vi "Mask and Limit Testing of XY Graph.vi"() -> ()   [LabVIEW 2023]
doc: "This example demonstrates how to create mask for XY graph. The VI checks if the input signal points are in or out of boundary. If any input signal points go beyond boundary, they will be marked in red. You can modify the boundary points that define a polygon and reset them."
uses:
  <vilib>/Analysis/NI_AALBase.lvlib
panel:
  out "XY Graph":cluster{"X":dbl[], "Y":dbl[]}[](graph)
  in  "Boundary":cluster{"X":dbl[], "Y":dbl[]}={"X"=[-0.6, 0.2, 1.0, 0.6, 0.0, -1.0], "Y"=[-1.0, -0.4, -0.6, 1.0, 0.4, 0.8]}
  in  "Reset Boundary":bool
  in  "stop":bool
  # "Overview: Demonstrates how to create a mask for an XY Graph. \nRequirements: LabVIEW Full Development System\nInstructions: \n1. Run the VI.\n2. Insert, delete or modify the boundary points. Click Reset Boundary to reset them.\n3. Click Stop to stop the VI."
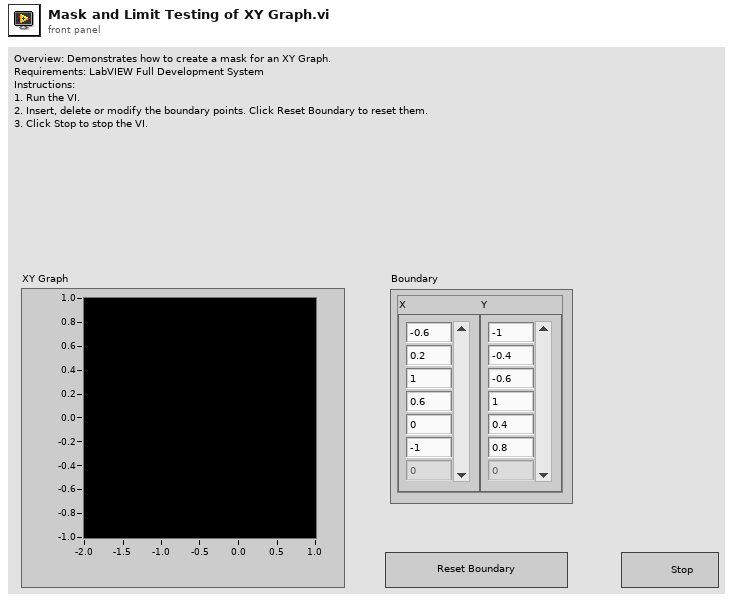
[diagram p1: front panel]
types:
  T1 = cluster{"Sinusoidal Pattern":dbl[], "Sinusoidal Pattern":dbl[]}
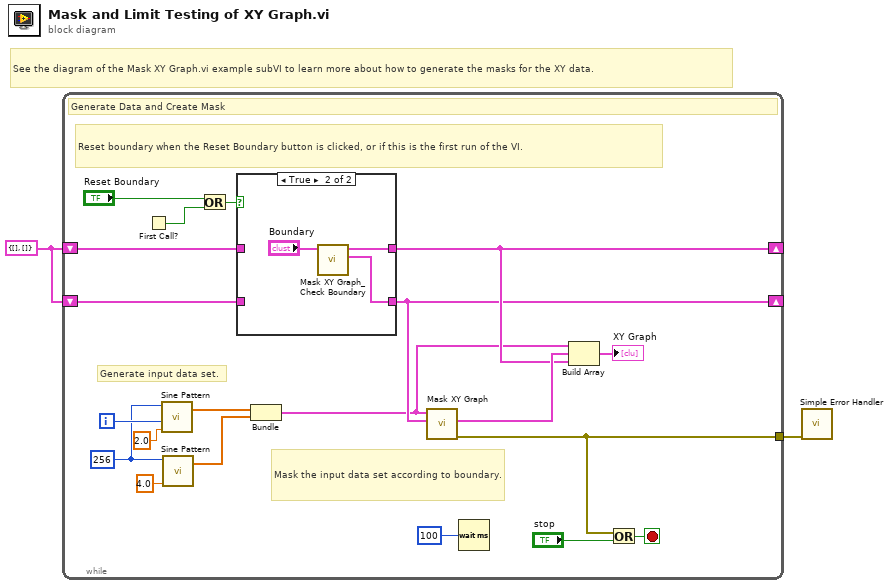
[diagram p0: block diagram]
diagram:
  w1 = cluster{"X":dbl[], "Y":dbl[]} {"X"=[], "Y"=[]} ("Closed Boundary")
  # "See the diagram of the Mask XY Graph.vi example subVI to learn more about how to generate the masks for the XY data."
  n1 = while {
    shift-right: [w17] -> _
    shift-left: w1 -> [w20]
    shift-right: [w16] -> _
    shift-left: w1 -> [w15]
    tunnel: [w5] -> w2
    i -> [w12]
    stop <- w6 stop-if-true
    w9 = 256 ("samples")
    # "Reset boundary when the Reset Boundary button is clicked, or if this is the first run of the VI."
    # "Mask the input data set according to boundary."
    # "Generate input data set."
    # "Generate Data and Create Mask"
    n2 = First Call?() -> (First Call?: T/F=w3:bool)
    n3 = call <vilib>:"Sine Pattern.vi"("cycles"=2.0, "phase(degrees)"=w12, "samples"=w9) -> ("Sinusoidal Pattern"=w11:dbl[])  [unwired: 1 in, 1 out]
    n4 = call <vilib>:"Sine Pattern.vi"("cycles"=4.0, "samples"=w9) -> ("Sinusoidal Pattern"=w10:dbl[])  [unwired: 2 in, 1 out]
    n5 = Or(x="Reset Boundary", y=w3) -> (x .or. y?=w4:bool)
    n6 = case shown="True" w4 {
      tunnel: w20 -> [w24 _]
      tunnel: [w23 w25] -> w16
      tunnel: [w24 w26] -> w17
      tunnel: w15 -> [w23 _]
      frame False {
      }
      frame True {
        n7 = call "Mask XY Graph_Check Boundary.vi"("Boundary"="Boundary") -> ("Open Boundary"=w25:cluster{"X":dbl[], "Y":dbl[]}, "Closed Boundary"=w26:cluster{"X":dbl[], "Y":dbl[]})  [unwired: 9 in]
      }
    }
    n8 = Bundle("Sinusoidal Pattern"=w11, "Sinusoidal Pattern"=w10) -> (w7:T1)  [unwired: 1 in]
    n9 = call "Mask XY Graph.vi"("Mask"=w16, "Data"=w7) -> ("error out"=w5:errorcluster, "Unmasked Data"=w22:cluster{"X":dbl[], "Y":dbl[]})  [unwired: 1 in, 7 out]
    n10 = Wait (ms)(milliseconds to wait=u32 100) -> ()  [unwired: 1 out]
    n11 = Build Array(w7, w22, w17) -> (→"XY Graph":cluster{"X":dbl[], "Y":dbl[]}[])
    n12 = Or(x=w5, y="stop") -> (x .or. y?=w6:bool)
  }
  n13 = call <vilib>:"Simple Error Handler.vi"("error in (no error)"=w2) -> ()  [unwired: 4 in, 5 out]
